vi "Build Image Histogram with Options.vi"(6 "Update needed":bool, 8 "error in (no error)":errorcluster, 10 "Histogram Options":T2 {"Max Histogram Size" format="%.0e"}, 11 "Image in":T5) -> (0 "error out":errorcluster, 1 "Array Statistics":T1, 2 "Location of Maximum":dbl, 3 "Histogram":cluster{"Axis":dbl[], "Histogram":dbl[]})   [LabVIEW 2021, in "Image.lvlib"]
uses:
  Image.lvlib
  <vilib>/vision/Image Controls.llb/IMAQ Image.ctl
  Histograms/Linear Histogram Options.ctl
  Histograms/Histogram Bin Option.ctl
  Histograms/Histogram Bin Position.ctl
  Arrays/Array Statistics.ctl
  5d79fc1d-7772-4591-8273-c1a574f3a5b5.vi
  73ce97dc-09df-4b78-8de3-323a3c338e66.vi
  03e3a8f1-a639-487f-9520-15d61c8637ec.vi
  0a471f91-9566-4d35-b541-cb4c4410c383.vi
  5d79fc1d-7772-4591-8273-c1a574f3a5b5.vi/e021cd17-e000-4244-b7f4-ec50548bdfcb.vi
  5d79fc1d-7772-4591-8273-c1a574f3a5b5.vi/b1828c6e-eb0a-43e9-a724-8b596c52e435.vi
  5d79fc1d-7772-4591-8273-c1a574f3a5b5.vi/be410ed7-52bf-46cf-99b8-7f99ae1f03fb.vi
  5d79fc1d-7772-4591-8273-c1a574f3a5b5.vi/52c6b4fa-501b-4af0-803b-8bab516ca5d3.vi
  5d79fc1d-7772-4591-8273-c1a574f3a5b5.vi/d7237e10-35ab-4bcb-a0c6-4883c3f4c990.vi
  5d79fc1d-7772-4591-8273-c1a574f3a5b5.vi/5fb5dd96-3b97-4592-ba56-58181c8e7105.vi
  5d79fc1d-7772-4591-8273-c1a574f3a5b5.vi/8e13a849-a393-4484-9968-4af7b25c38d7.vi
  73ce97dc-09df-4b78-8de3-323a3c338e66.vi/e021cd17-e000-4244-b7f4-ec50548bdfcb.vi
  73ce97dc-09df-4b78-8de3-323a3c338e66.vi/b1828c6e-eb0a-43e9-a724-8b596c52e435.vi
  73ce97dc-09df-4b78-8de3-323a3c338e66.vi/be410ed7-52bf-46cf-99b8-7f99ae1f03fb.vi
  73ce97dc-09df-4b78-8de3-323a3c338e66.vi/52c6b4fa-501b-4af0-803b-8bab516ca5d3.vi
  73ce97dc-09df-4b78-8de3-323a3c338e66.vi/d7237e10-35ab-4bcb-a0c6-4883c3f4c990.vi
  73ce97dc-09df-4b78-8de3-323a3c338e66.vi/5fb5dd96-3b97-4592-ba56-58181c8e7105.vi
  73ce97dc-09df-4b78-8de3-323a3c338e66.vi/8e13a849-a393-4484-9968-4af7b25c38d7.vi
  03e3a8f1-a639-487f-9520-15d61c8637ec.vi/e021cd17-e000-4244-b7f4-ec50548bdfcb.vi
  03e3a8f1-a639-487f-9520-15d61c8637ec.vi/b1828c6e-eb0a-43e9-a724-8b596c52e435.vi
  03e3a8f1-a639-487f-9520-15d61c8637ec.vi/7a6138ed-c001-4311-b538-9ba42ae7c7b1.vi
  03e3a8f1-a639-487f-9520-15d61c8637ec.vi/52c6b4fa-501b-4af0-803b-8bab516ca5d3.vi
  03e3a8f1-a639-487f-9520-15d61c8637ec.vi/d7237e10-35ab-4bcb-a0c6-4883c3f4c990.vi
  03e3a8f1-a639-487f-9520-15d61c8637ec.vi/5fb5dd96-3b97-4592-ba56-58181c8e7105.vi
  03e3a8f1-a639-487f-9520-15d61c8637ec.vi/8e13a849-a393-4484-9968-4af7b25c38d7.vi
  0a471f91-9566-4d35-b541-cb4c4410c383.vi/e021cd17-e000-4244-b7f4-ec50548bdfcb.vi
  0a471f91-9566-4d35-b541-cb4c4410c383.vi/b1828c6e-eb0a-43e9-a724-8b596c52e435.vi
  0a471f91-9566-4d35-b541-cb4c4410c383.vi/be410ed7-52bf-46cf-99b8-7f99ae1f03fb.vi
  0a471f91-9566-4d35-b541-cb4c4410c383.vi/52c6b4fa-501b-4af0-803b-8bab516ca5d3.vi
  0a471f91-9566-4d35-b541-cb4c4410c383.vi/d7237e10-35ab-4bcb-a0c6-4883c3f4c990.vi
  0a471f91-9566-4d35-b541-cb4c4410c383.vi/5fb5dd96-3b97-4592-ba56-58181c8e7105.vi
  0a471f91-9566-4d35-b541-cb4c4410c383.vi/8e13a849-a393-4484-9968-4af7b25c38d7.vi
  <vilib>/vision/EDVR.llb/IMAQ ImageToEDVR 2D U8.vi
  Time/High Resolution Timing.vi
  <vilib>/Utility/error.llb/Error Cluster From Error Code.vi
  <vilib>/vision/EDVR.llb/IMAQ ImageToEDVR 2D I16.vi
  <vilib>/vision/EDVR.llb/IMAQ ImageToEDVR 2D SGL.vi
  <userlib>/_OpenG.lib/array/array.llb/Filter 1D Array__ogtk.vi
  <userlib>/_OpenG.lib/array/array.llb/Filter 1D Array (SGL)__ogtk.vi
  <userlib>/_OpenG.lib/array/array.llb/Delete Elements from Array__ogtk.vi
  <userlib>/_OpenG.lib/array/array.llb/Delete Elements from 1D Array (DBL)__ogtk.vi
  <vilib>/vision/EDVR.llb/IMAQ ImageToEDVR 2D U16.vi
  <vilib>/ErrorRing/Error Ring.xnode
  Histograms/Histogram Window.lvlib
  Arrays/Arrays.lvlib
panel:
  in  "# Bins":i32
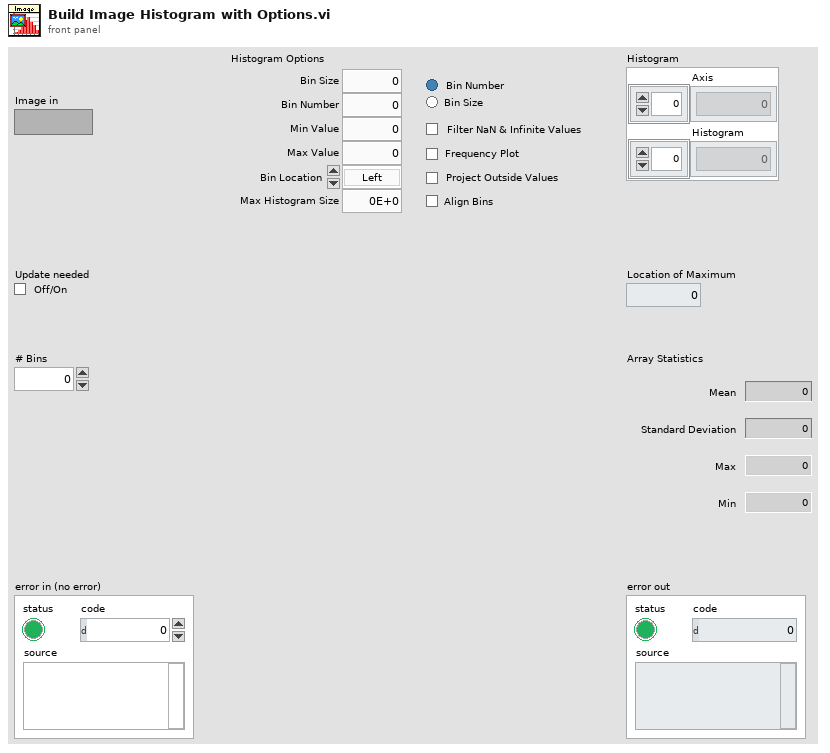
[diagram p1: front panel]
types:
  T1 = typedef "Arrays.lvlib/Array Statistics.ctl" = cluster{"Mean":dbl, "Standard Deviation":dbl, "Max":dbl, "Min":dbl}
  T2 = typedef "Histogram Window.lvlib/Linear Histogram Options.ctl" = cluster{"Bin Size":dbl, "Bin Number":i32, "Bin Option":T3, "Min Value":dbl, "Max Value":dbl, "Filter NaN & Infinite Values":bool, "Frequency Plot":bool, "Align Bins":bool, "Bin Location":T4, "Project Outside Values":bool, "Max Histogram Size":i32}
  T3 = typedef "Histogram Window.lvlib/Histogram Bin Option.ctl" = enum32{"Bin Number", "Bin Size"}
  T4 = typedef "Histogram Window.lvlib/Histogram Bin Position.ctl" = enum16{"Left", "Center", "Right"}
  T5 = typedef "IMAQ Image.ctl" = refnum<image>
  T6 = typedef "Image Type" = u32
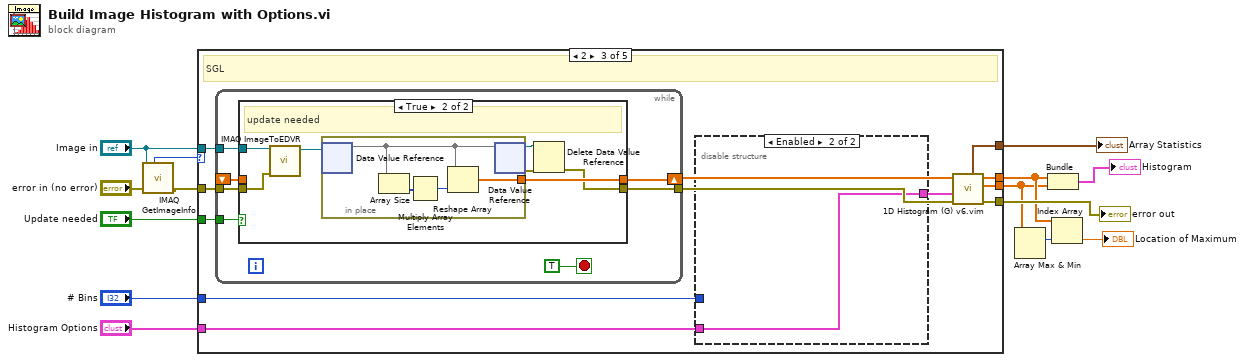
[diagram p0: block diagram]
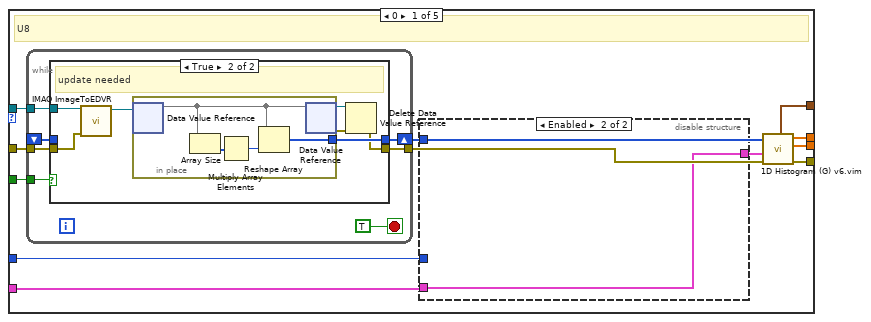
[diagram p2: hidden frame]
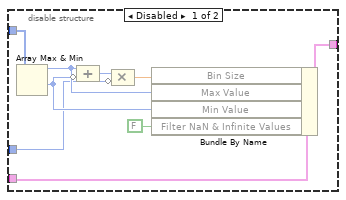
[diagram p3: hidden frame]
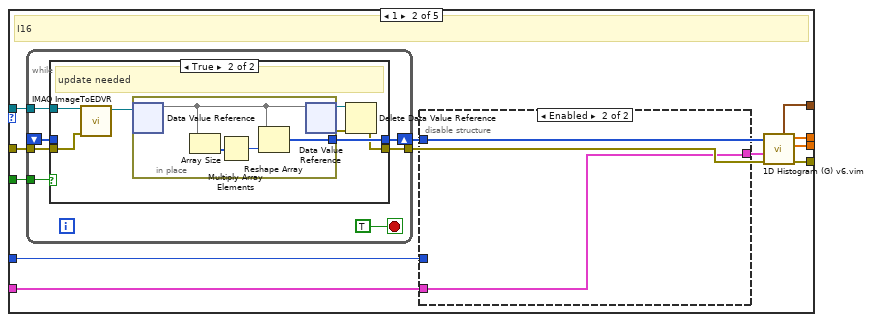
[diagram p5: hidden frame]
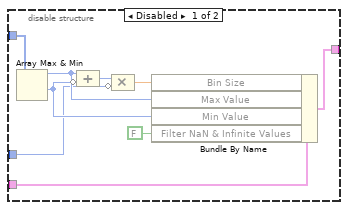
[diagram p6: hidden frame]
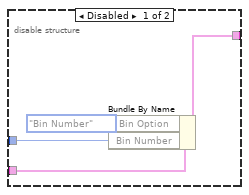
[diagram p8: hidden frame]
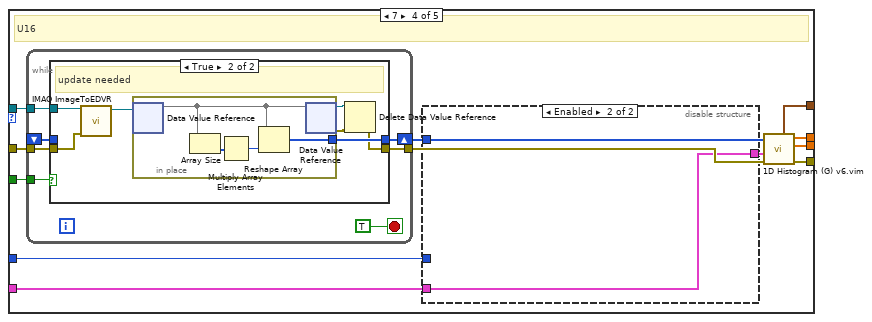
[diagram p10: hidden frame]
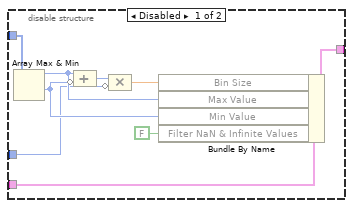
[diagram p11: hidden frame]
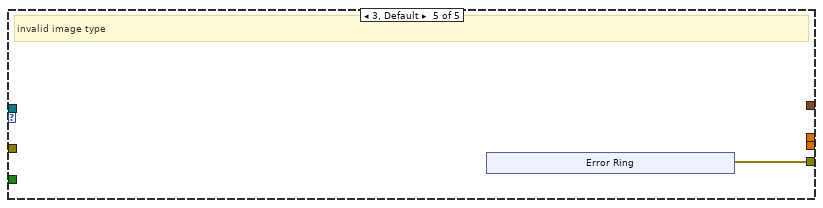
[diagram p13: hidden frame]
diagram:
  n1 = call "IMAQ GetImageInfo"("error in (no error)"="error in (no error)", "Image"="Image in") -> ("error out"=w13:errorcluster, "Image Type"=w12:T6)  [unwired: 2 in, 6 out]
  n2 = case shown="2" w12 {
    tunnel: w13 -> [w25 w67 w109 w146 _]
    tunnel: "Image in" -> [w26 w68 w110 w147 _]
    tunnel: [w22 w63 w105 w142 _] -> w2
    tunnel: [w23 w64 w106 w143 _] -> w1
    tunnel: [w24 w65 w107 w144 w178] -> w9
    tunnel: "Histogram Options" -> [w17 w62 w102 w141 _]
    tunnel: "# Bins" -> [w20 w60 w100 w139 _]
    tunnel: [w15 w57 w99 w136 _] -> w7
    tunnel: "Update needed" -> [w18 w58 w104 w137 _]
    frame 0 {
      # "U8"
      n3 = while {
        tunnel: w26 -> [w43]
        tunnel: w25 -> [w42]
        tunnel: [w41] -> w16
        shift-right: [w40] -> w19
        shift-left: _ -> [w38]
        tunnel: w18 -> [w37]
        stop <- TRUE stop-if-true
        n4 = case shown="True" w37 {
          tunnel: w43 -> [_ w52]
          tunnel: w42 -> [w45 w51]
          tunnel: [w45 w46] -> w41
          tunnel: [w44 w49] -> w40
          tunnel: w38 -> [w44 _]
          frame False {
            # "no update needed"
          }
          frame True {
            # "update needed"
            n5 = call-poly <vilib>:"IMAQ ImageToEDVR.vi"("error in (no error)"=w51, "Image"=w52) -> ("EDVR 2D U8"=w50:refnum<data-value>)  [unwired: 7 in, 2 out]
            n6 = in-place {
              in-place-border: [w54] -> w49
              n7 = in-place-dvr #1(w50) -> (w53:u8[][])  [unwired: 1 out]
              n8 = Array Size(array=w53) -> (size(s)=w56:i32[])
              n9 = Multiply Array Elements(1:w56) -> (0:w55:i32)
              n10 = Reshape Array(w53, w55) -> (w54:u8[])
              n11 = in-place-dvr #1(w53) -> (w48:refnum<data-value>, w47:errorcluster)
            }
            n12 = Delete Data Value Reference(data value reference=w48, error in=w47) -> (error out=w46:errorcluster)  [unwired: 1 out]
          }
        }
      }
      n13 = disable-structure shown="Enabled" {
        disable-tunnel: [w35 w36] -> w21
        disable-tunnel: w20 -> [w31 _]
        disable-tunnel: w19 -> [w30 _]
        disable-tunnel: w17 -> [w28 w36]
        frame Disabled {
          n14 = Array Max & Min(array=w30) -> (max value=w33:u8, min value=w34:u8)  [unwired: 2 out]
          n15 = Compound Arithmetic op=ADD(w33, invert w34) -> (w32:u8)
          n16 = Compound Arithmetic op=MULTIPLY(w32, invert w31) -> (w29:dbl)
          n17 = Bundle By Name(cluster=w28, "Bin Size"=w29, "Max Value"=w33, "Min Value"=w34, "Filter NaN & Infinite Values"=FALSE) -> (w35:T2)
        }
        frame Enabled {
        }
      }
      n18 = call "1D Histogram (G) v6.vim"("Error In"=w16, "Histogram Options"=w21, "Array"=w19) -> ("Error Out"=w24:errorcluster, "Histogram"=w23:dbl[], "Axis"=w22:dbl[], "Array Statistics"=w15:T1)  [unwired: 2 in, 3 out]
    }
    frame 1 {
      # "I16"
      n19 = while {
        tunnel: w68 -> [w85]
        tunnel: w67 -> [w84]
        tunnel: [w83] -> w66
        shift-right: [w82] -> w59
        shift-left: _ -> [w80]
        tunnel: w58 -> [w79]
        stop <- TRUE stop-if-true
        n20 = case shown="True" w79 {
          tunnel: w85 -> [_ w94]
          tunnel: w84 -> [w87 w93]
          tunnel: [w87 w88] -> w83
          tunnel: [w86 w91] -> w82
          tunnel: w80 -> [w86 _]
          frame False {
            # "no update needed"
          }
          frame True {
            # "update needed"
            n21 = call-poly <vilib>:"IMAQ ImageToEDVR.vi"("error in (no error)"=w93, "Image"=w94) -> ("EDVR 2D I16"=w92:refnum<data-value>)  [unwired: 7 in, 2 out]
            n22 = in-place {
              in-place-border: [w96] -> w91
              n23 = in-place-dvr #2(w92) -> (w95:i16[][])  [unwired: 1 out]
              n24 = Array Size(array=w95) -> (size(s)=w98:i32[])
              n25 = Multiply Array Elements(1:w98) -> (0:w97:i32)
              n26 = Reshape Array(w95, w97) -> (w96:i16[])
              n27 = in-place-dvr #2(w95) -> (w90:refnum<data-value>, w89:errorcluster)
            }
            n28 = Delete Data Value Reference(data value reference=w90, error in=w89) -> (error out=w88:errorcluster)  [unwired: 1 out]
          }
        }
      }
      n29 = disable-structure shown="Enabled" {
        disable-tunnel: w62 -> [w77 w78]
        disable-tunnel: [w76 w78] -> w61
        disable-tunnel: w60 -> [w72 _]
        disable-tunnel: w59 -> [w71 _]
        frame Disabled {
          n30 = Array Max & Min(array=w71) -> (max value=w74:i16, min value=w75:i16)  [unwired: 2 out]
          n31 = Compound Arithmetic op=ADD(w74, invert w75) -> (w73:i16)
          n32 = Compound Arithmetic op=MULTIPLY(w73, invert w72) -> (w70:dbl)
          n33 = Bundle By Name(cluster=w77, "Bin Size"=w70, "Max Value"=w74, "Min Value"=w75, "Filter NaN & Infinite Values"=FALSE) -> (w76:T2)
        }
        frame Enabled {
        }
      }
      n34 = call "1D Histogram (G) v6.vim"("Error In"=w66, "Histogram Options"=w61, "Array"=w59) -> ("Error Out"=w65:errorcluster, "Histogram"=w64:dbl[], "Axis"=w63:dbl[], "Array Statistics"=w57:T1)  [unwired: 2 in, 3 out]
    }
    frame 2 {
      # "SGL"
      n35 = while {
        tunnel: w110 -> [w122]
        tunnel: w109 -> [w121]
        tunnel: [w120] -> w108
        shift-right: [w119] -> w103
        shift-left: _ -> [w117]
        tunnel: w104 -> [w116]
        stop <- TRUE stop-if-true
        n36 = case shown="True" w116 {
          tunnel: w122 -> [_ w131]
          tunnel: w121 -> [w124 w130]
          tunnel: [w124 w125] -> w120
          tunnel: [w123 w128] -> w119
          tunnel: w117 -> [w123 _]
          frame False {
            # "no update needed"
          }
          frame True {
            # "update needed"
            n37 = call-poly <vilib>:"IMAQ ImageToEDVR.vi"("error in (no error)"=w130, "Image"=w131) -> ("EDVR 2D SGL"=w129:refnum<data-value>)  [unwired: 7 in, 2 out]
            n38 = in-place {
              in-place-border: [w133] -> w128
              n39 = in-place-dvr #3(w129) -> (w132:sgl[][])  [unwired: 1 out]
              n40 = Array Size(array=w132) -> (size(s)=w135:i32[])
              n41 = Multiply Array Elements(1:w135) -> (0:w134:i32)
              n42 = Reshape Array(w132, w134) -> (w133:sgl[])
              n43 = in-place-dvr #3(w132) -> (w127:refnum<data-value>, w126:errorcluster)
            }
            n44 = Delete Data Value Reference(data value reference=w127, error in=w126) -> (error out=w125:errorcluster)  [unwired: 1 out]
          }
        }
      }
      n45 = disable-structure shown="Enabled" {
        disable-tunnel: w102 -> [w114 w115]
        disable-tunnel: [w113 w115] -> w101
        disable-tunnel: w100 -> [w112 _]
        frame Disabled {
          n46 = Bundle By Name(cluster=w114, "Bin Option"=Histogram_Bin_Option."Bin Number", "Bin Number"=w112) -> (w113:T2)
        }
        frame Enabled {
        }
      }
      n47 = call "1D Histogram (G) v6.vim"("Error In"=w108, "Histogram Options"=w101, "Array"=w103) -> ("Error Out"=w107:errorcluster, "Histogram"=w106:dbl[], "Axis"=w105:dbl[], "Array Statistics"=w99:T1)  [unwired: 2 in, 3 out]
    }
    frame 7 {
      # "U16"
      n48 = while {
        tunnel: w147 -> [w164]
        tunnel: w146 -> [w163]
        tunnel: [w162] -> w145
        shift-right: [w161] -> w138
        shift-left: _ -> [w159]
        tunnel: w137 -> [w158]
        stop <- TRUE stop-if-true
        n49 = case shown="True" w158 {
          tunnel: w164 -> [_ w173]
          tunnel: w163 -> [w166 w172]
          tunnel: [w166 w167] -> w162
          tunnel: [w165 w170] -> w161
          tunnel: w159 -> [w165 _]
          frame False {
            # "no update needed"
          }
          frame True {
            # "update needed"
            n50 = call-poly <vilib>:"IMAQ ImageToEDVR.vi"("error out"=w172, "Image"=w173) -> ("EDVR 2D U16"=w171:refnum<data-value>)  [unwired: 7 in, 2 out]
            n51 = in-place {
              in-place-border: [w175] -> w170
              n52 = in-place-dvr #4(w171) -> (w174:u16[][])  [unwired: 1 out]
              n53 = Array Size(array=w174) -> (size(s)=w177:i32[])
              n54 = Multiply Array Elements(1:w177) -> (0:w176:i32)
              n55 = Reshape Array(w174, w176) -> (w175:u16[])
              n56 = in-place-dvr #4(w174) -> (w169:refnum<data-value>, w168:errorcluster)
            }
            n57 = Delete Data Value Reference(data value reference=w169, error in=w168) -> (error out=w167:errorcluster)  [unwired: 1 out]
          }
        }
      }
      n58 = disable-structure shown="Enabled" {
        disable-tunnel: w141 -> [w156 w157]
        disable-tunnel: [w155 w157] -> w140
        disable-tunnel: w139 -> [w151 _]
        disable-tunnel: w138 -> [w150 _]
        frame Disabled {
          n59 = Array Max & Min(array=w150) -> (max value=w153:u16, min value=w154:u16)  [unwired: 2 out]
          n60 = Compound Arithmetic op=ADD(w153, invert w154) -> (w152:u16)
          n61 = Compound Arithmetic op=MULTIPLY(w152, invert w151) -> (w149:dbl)
          n62 = Bundle By Name(cluster=w156, "Bin Size"=w149, "Max Value"=w153, "Min Value"=w154, "Filter NaN & Infinite Values"=FALSE) -> (w155:T2)
        }
        frame Enabled {
        }
      }
      n63 = call "1D Histogram (G) v6.vim"("Error In"=w145, "Histogram Options"=w140, "Array"=w138) -> ("Error Out"=w144:errorcluster, "Histogram"=w143:dbl[], "Axis"=w142:dbl[], "Array Statistics"=w136:T1)  [unwired: 2 in, 3 out]
    }
    frame 3, Default {
      # "invalid image type"
      n64 = xnode "Error Ring"() -> ("error out"=w178:errorcluster)
    }
  }
  "error out" <- w9
  "Array Statistics" <- w7
  n65 = Array Max & Min(array=w1) -> (max index (indices)=w3:i32)  [unwired: 3 out]
  n66 = Bundle("Axis"=w2, "Histogram"=w1) -> (→"Histogram":cluster{"Axis":dbl[], "Histogram":dbl[]})  [unwired: 1 in]
  n67 = Index Array(array=w2, index=w3) -> (element=→"Location of Maximum":dbl)
